vi "Remove Unselected Channels_Detectors_Objectives from XML Object.vi"(8 "error in (no error)":errorcluster, 11 "Document Refnum IN":refnum<k20>) -> (0 "error out":errorcluster, 3 "Document Refnum Out":refnum<k20>)   [LabVIEW 2012]
doc: "SciScan 1.2 160622"
uses:
  GFG/GFG library.lvlib
  <vilib>/xml/NI_XML.lvlib
  <resource>/objmgr/DOMUserDefRef.rc
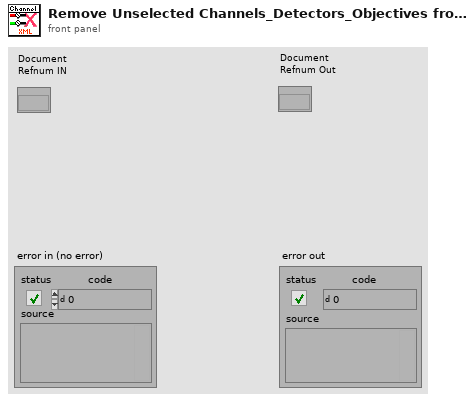
[diagram p1: front panel]
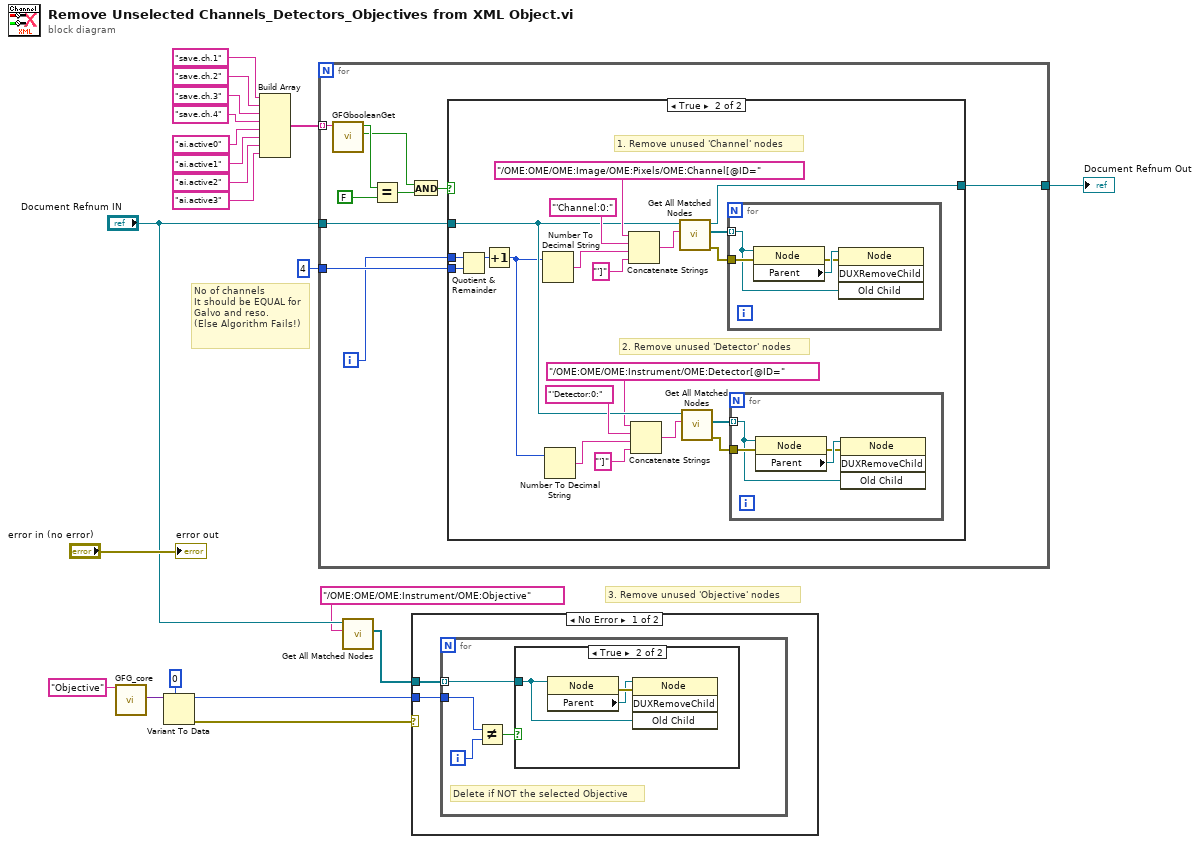
[diagram p0: block diagram]
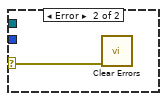
[diagram p3: hidden frame]
diagram:
  # "3. Remove unused 'Objective' nodes"
  # "No of channels\nIt should be EQUAL for Galvo and reso.\n(Else Algorithm Fails!)"
  n1 = call "GFG_core.vi"("Variable Name in"="Objective") -> ("Variant Out"=w7:variant)  [unwired: 12 in, 6 out]
  n2 = Variant To Data(type=u16 0 ("y"), Variant=w7) -> (data=w1:u16, error out=w3:errorcluster)  [unwired: 1 in]
  n3 = Build Array("save.ch.1" ("Variable Name in"), "save.ch.2" ("Variable Name in"), "save.ch.3" ("Variable Name in"), "save.ch.4" ("Variable Name in"), "ai.active0" ("Variable Name in"), "ai.active1" ("Variable Name in"), "ai.active2" ("Variable Name in"), "ai.active3" ("Variable Name in")) -> (w18:string[])
  n4 = for {
    tunnel: w18 -> [w30] mode=indexing
    tunnel: 4 ("y") -> [w29]
    tunnel: "Document Refnum IN" -> [w27]
    tunnel: [w26] -> w20
    i -> [w28]
    n5 = call "GFGbooleanGet.vi"("Variable Name in"=w30) -> ("Found/Replaced"=w21:bool, "Boolean Value OUT"=w25:bool)  [unwired: 9 in]
    n6 = Equal?(x=w25, y=FALSE) -> (x = y?=w22:bool)
    n7 = And(x=w21, y=w22) -> (x .and. y?=w23:bool)
    n8 = case shown="True" w23 {
      tunnel: w28 -> [_ w51]
      tunnel: w29 -> [_ w50]
      tunnel: w27 -> [w31 w34]
      tunnel: [w31 w45] -> w26
      frame False {
      }
      frame True {
        # "2. Remove unused 'Detector' nodes"
        # "1. Remove unused 'Channel' nodes"
        n9 = Quotient & Remainder(x=w51, y=w50) -> (x-y*floor(x/y)=w49:i32)  [unwired: 1 out]
        n10 = Increment(x=w49) -> (x+1=w32:i32)
        n11 = Number To Decimal String(number=w32) -> (decimal integer string=w42:string)  [unwired: 1 in]
        n12 = Number To Decimal String(number=w32) -> (decimal integer string=w39:string)  [unwired: 1 in]
        n13 = Concatenate Strings("/OME:OME/OME:Image/OME:Pixels/OME:Channel[@ID=" ("XPath expression"), "'Channel:0:" ("XPath expression"), w42, "']" ("XPath expression")) -> (w46:string)
        n14 = Concatenate Strings("/OME:OME/OME:Instrument/OME:Detector[@ID=" ("XPath expression"), "'Detector:0:" ("XPath expression"), w39, "']" ("XPath expression")) -> (w36:string)
        n15 = call <vilib>:"Get All Matched Nodes.vi"("XPath expression"=w46, "node in"=w34) -> ("error out"=w44:errorcluster, "node result array"=w43:refnum<k20>[], "node out"=w45:refnum<k20>)  [unwired: 7 in]
        n16 = call <vilib>:"Get All Matched Nodes.vi"("XPath expression"=w36, "node in"=w34) -> ("error out"=w37:errorcluster, "node result array"=w38:refnum<k20>[])  [unwired: 7 in, 1 out]
        n17 = for {
          tunnel: w44 -> [w57]
          tunnel: w43 -> [w56] mode=indexing
          n18 = property class="Node"(reference=w56, error in=w57) -> (error out=w58:errorcluster, "Parent"=w59:refnum<k20>)  [unwired: 1 out]
          n19 = invoke class="Node" method="DUXRemoveChild"(reference=w59, error in=w58, "Old Child"=w56) -> ()  [unwired: 1 in, 4 out]
        }
        n20 = for {
          tunnel: w37 -> [w53]
          tunnel: w38 -> [w52] mode=indexing
          n21 = property class="Node"(reference=w52, error in=w53) -> (error out=w54:errorcluster, "Parent"=w55:refnum<k20>)  [unwired: 1 out]
          n22 = invoke class="Node" method="DUXRemoveChild"(reference=w55, error in=w54, "Old Child"=w52) -> ()  [unwired: 1 in, 4 out]
        }
      }
    }
  }
  "Document Refnum Out" <- w20
  n23 = call <vilib>:"Get All Matched Nodes.vi"("XPath expression"="/OME:OME/OME:Instrument/OME:Objective", "node in"="Document Refnum IN") -> ("node result array"=w2:refnum<k20>[])  [unwired: 7 in, 2 out]
  n24 = case shown="No Error" w3 {
    selector: w3 -> [_ w69]
    tunnel: w2 -> [w61 _]
    tunnel: w1 -> [w60 _]
    frame No Error {
      n25 = for {
        tunnel: w61 -> [w62] mode=indexing
        tunnel: w60 -> [w64]
        i -> [w65]
        # "Delete if NOT the selected Objective"
        n26 = Not Equal?(x=w64, y=w65) -> (x != y?=w63:bool)
        n27 = case shown="True" w63 {
          tunnel: w62 -> [_ w66]
          frame False {
          }
          frame True {
            n28 = property class="Node"(reference=w66) -> (error out=w68:errorcluster, "Parent"=w67:refnum<k20>)  [unwired: 1 in, 1 out]
            n29 = invoke class="Node" method="DUXRemoveChild"(reference=w67, error in=w68, "Old Child"=w66) -> ()  [unwired: 1 in, 4 out]
          }
        }
      }
    }
    frame Error {
      n30 = call <vilib>:"Clear Errors.vi"("error in (no error)"=w69) -> ()  [unwired: 6 in, 1 out]
    }
  }
  "error out" <- "error in (no error)"
